vi "Config_flotas.vi"(8 "file path (dialog if empty)":path) -> (0 "Distancias generales":dbl[](array[numeric]), 1 "Puntos medios de las ventanas":dbl[][](array[numeric]), 2 "Distancia de acelerómetros":dbl[](array[numeric]), 3 "Distacias y medidas de dispositivos":bool=TRUE, 4 "Series_flota":string[](array[string]))   [LabVIEW 2015]
panel:
  out "text":string
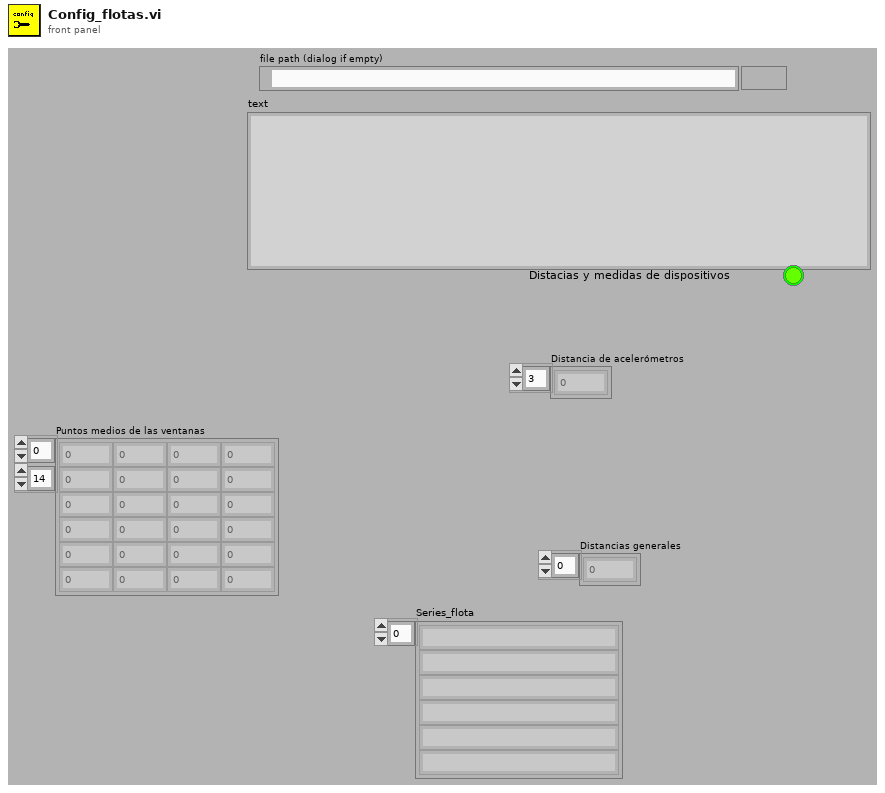
[diagram p1: front panel]
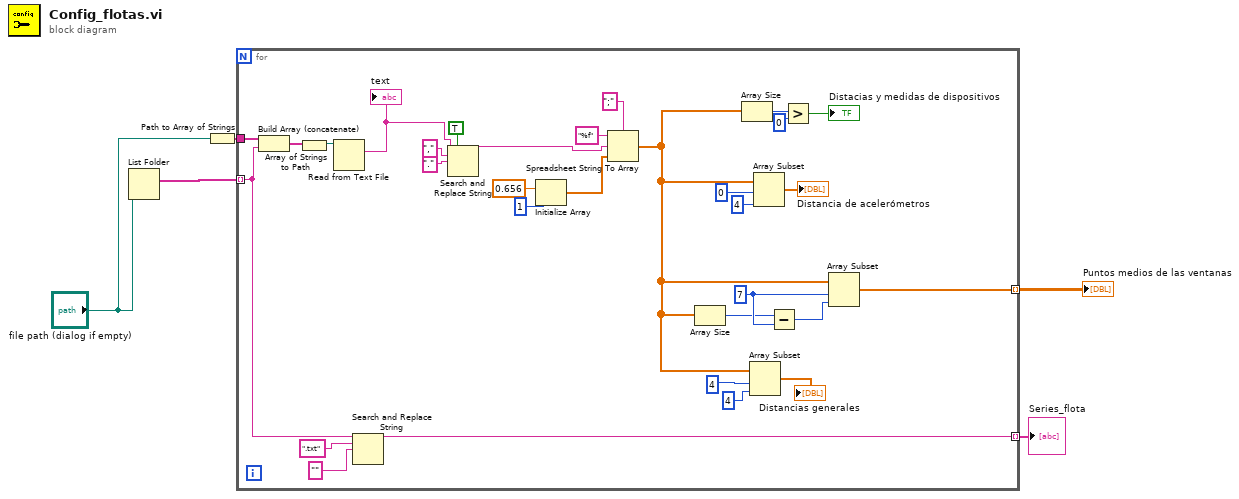
[diagram p0: block diagram]
diagram:
  n1 = List Folder(path="file path (dialog if empty)") -> (filenames=w3:string[])  [unwired: 3 in, 3 out]
  n2 = Path to Array of Strings(0:"file path (dialog if empty)") -> (2:w4:string[])  [unwired: 1 out]
  n3 = for {
    tunnel: w4 -> [w18]
    tunnel: w3 -> [w12] mode=indexing
    tunnel: [w15] -> w2 mode=indexing
    tunnel: [w11] -> w1 mode=indexing
    w24 = 7 ("index")
    n4 = Build Array (concatenate)(w18, w12) -> (w17:string[])
    n5 = Array of Strings to Path(0:w17) -> (2:w16:path)  [unwired: 1 out]
    n6 = Read from Text File(file (use dialog)=w16) -> (text=w7:string)  [unwired: 3 in, 3 out]
    "text" <- w7
    n7 = Search and Replace String(input string=w12, search string=".txt" ("substring (\"\")"), replace string="" ("substring (\"\")")) -> (result string=w11:string)  [unwired: 5 in, 3 out]
    n8 = Search and Replace String(replace all?=TRUE ("replace all? (F)"), input string=w7, search string=",", replace string="." ("replace string (\"\")")) -> (result string=w6:string)  [unwired: 4 in, 3 out]
    n9 = Initialize Array(0.656 ("element"), 1 ("dimension size")) -> (w32:dbl[])
    n10 = Spreadsheet String To Array(delimiter (Tab)=";" ("prompt (Open existing file)"), format string="%f", spreadsheet string=w6, array type (2D Dbl)=w32) -> (array=w19:dbl[])
    n11 = Array Size(array=w19) -> (size(s)=w23:i32)
    n12 = Array Size(array=w19) -> (size(s)=w31:i32)
    n13 = Array Subset(array=w19, index=4, length=4) -> (→"Distancias generales":dbl[])
    n14 = Array Subset(array=w19, index=0, length=4) -> (→"Distancia de acelerómetros":dbl[])
    n15 = Subtract(x=w23, y=w24) -> (x-y=w25:i32)
    n16 = Greater?(x=w31, y=0) -> (0:→"Distacias y medidas de dispositivos":bool)
    n17 = Array Subset(array=w19, index=w24, length=w25) -> (w15:dbl[])
  }
  "Puntos medios de las ventanas" <- w2
  "Series_flota" <- w1
